vi "串口打开状况界面操作.vi"(6 "布尔":bool, 7 "选项":enum16{"初始化", "操作"}(ring), 8 "错误输入（无错误）":errorcluster, 9 "数组":string[](array[string]), 10 "本VI":refnum<vi>, 11 "Boolean输入":refnum<vi>) -> (0 "error out":errorcluster, 3 "Controls[]":refnum<vi>[](array[refnum]))   [LabVIEW 2017]
panel:
  out "已删除控件":refnum<vi>[](array[refnum])
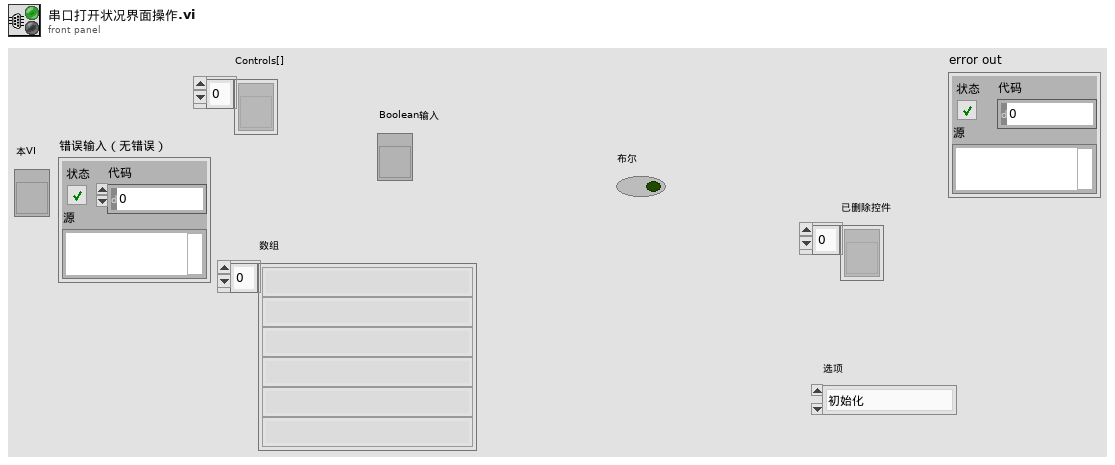
[diagram p1: front panel]
types:
  T1 = enum8{"Enabled", "Disabled", "Disabled and Grayed Out"}
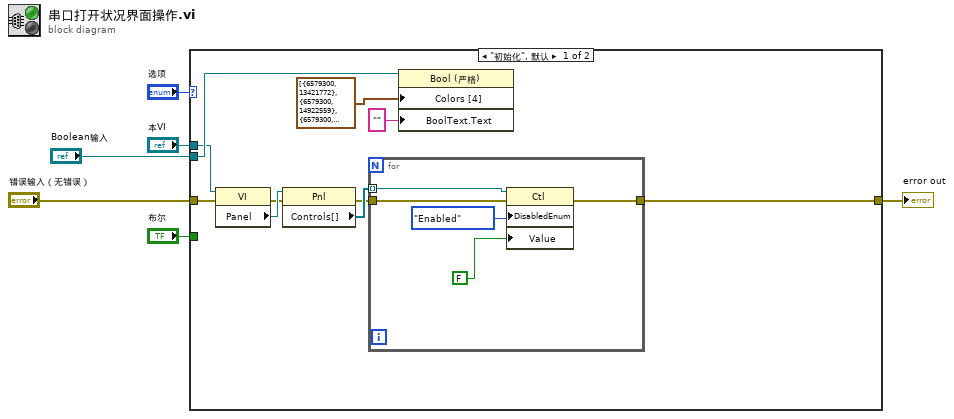
[diagram p0: block diagram]
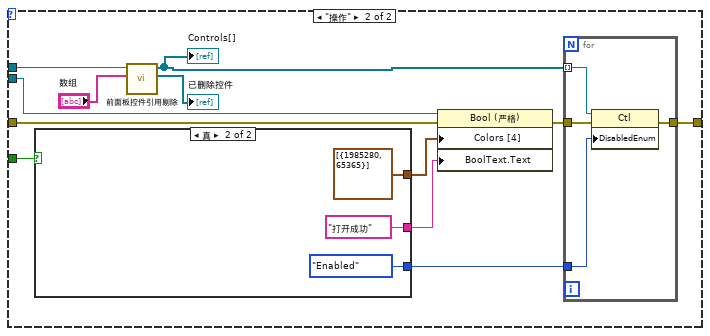
[diagram p2: hidden frame]
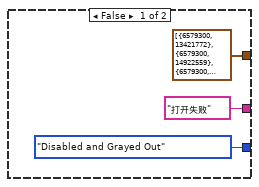
[diagram p3: hidden frame]
diagram:
  n1 = case shown="\"初始化\", 默认" "选项" {
    tunnel: "本VI" -> [w12 w31]
    tunnel: "Boolean输入" -> [w16 w26]
    tunnel: "布尔" -> [_ w25]
    tunnel: [w7 w23] -> w1
    tunnel: "错误输入（无错误）" -> [w10 w22]
    frame "初始化", Default {
      n2 = property on="属性节点" class="VI"(reference=w12, error in=w10) -> (error out=w9:errorcluster, "Panel"=w13:refnum<vi>)  [unwired: 1 out]
      n3 = property on="属性节点" class="Pnl"(reference=w13, error in=w9) -> (error out=w8:errorcluster, "Controls[]"=w11:refnum<vi>[])  [unwired: 1 out]
      n4 = for {
        tunnel: w11 -> [w21] mode=indexing
        tunnel: w8 -> [w19]
        tunnel: [w18] -> w7
        n5 = property class="Ctl"(reference=w21, error in=w19, "DisabledEnum"=T1."Enabled" ("禁用"), "Value"=FALSE) -> (error out=w18:errorcluster)  [unwired: 1 out]
      }
      n6 = property class="Bool (严格)"(reference=w16, "Colors [4]"=cluster{u32, u32}[] [{6579300, 13421772}, {6579300, 14922559}, {6579300, 13421772}, {6579300, 14922559}] ("颜色[4]"), "BoolText.Text"="" ("布尔文本.文本")) -> ()  [unwired: 1 in, 2 out]
    }
    frame "操作" {
      n7 = case shown="真" w25 {
        tunnel: [T1."Disabled and Grayed Out" ("禁用") T1."Enabled" ("禁用")] -> w30
        tunnel: [cluster{u32, u32}[] [{6579300, 13421772}, {6579300, 14922559}, {6579300, 13421772}, {6579300, 14922559}] ("颜色[4]") cluster{u32, u32}[] [{1985280, 65365}] ("颜色[4]")] -> w32
        tunnel: ["打开失败" ("布尔文本.文本") "打开成功" ("布尔文本.文本")] -> w33
        frame False {
        }
        frame True {
        }
      }
      n8 = call "前面板控件引用剔除.vi"("数组"="数组", "VI输入"=w31) -> ("已删除控件"=→"已删除控件":refnum<vi>[], "删除后控件"=w29:refnum<vi>[])  [unwired: 8 in]
      "Controls[]" <- w29
      n9 = property class="Bool (严格)"(reference=w26, error in=w22, "Colors [4]"=w32, "BoolText.Text"=w33) -> (error out=w24:errorcluster)  [unwired: 1 out]
      n10 = for {
        tunnel: w29 -> [w43] mode=indexing
        tunnel: w30 -> [w42]
        tunnel: w24 -> [w41]
        tunnel: [w40] -> w23
        n11 = property class="Ctl"(reference=w43, error in=w41, "DisabledEnum"=w42) -> (error out=w40:errorcluster)  [unwired: 1 out]
      }
    }
  }
  "error out" <- w1
